vi "导入模版文件.vi"(8 "功率控制表":refnum<vi>, 9 "标定参数表":refnum<vi>, 11 "该应用程序":refnum<vi>) -> ()   [LabVIEW 2015]
uses:
  <vilib>/addons/_office/excel.llb/Excel Get Data ([str]).vi
  <vilib>/Utility/NIReport.llb/NI_report.lvclass
  <vilib>/Utility/NIReport.llb/Excel/NI_Excel.lvclass
  <vilib>/addons/_office/NI_ReportGenerationToolkit.lvlib
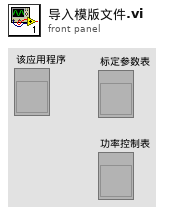
[diagram p1: front panel]
types:
  T1 = enum16{"Standard Report", "HTML", "Word", "Excel"}
  T2 = enum16{"maximized", "minimized", "normal", "no change"}
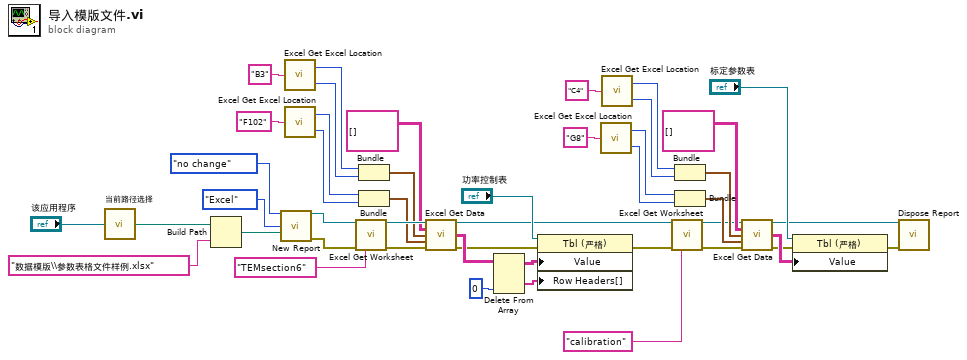
[diagram p0: block diagram]
diagram:
  n1 = call "当前路径选择.vi"("本应用程序"="该应用程序") -> ("当前路径"=w29:path)
  n2 = Build Path(base path=w29, name or relative path="数据模版\\参数表格文件样例.xlsx" ("名称或相对路径")) -> (appended path=w28:path)
  n3 = call <vilib>:"New Report.vi"("window state (normal)"=T2."no change", "report type"=T1."Excel", "template (empty)"=w28) -> ("report out"=w27:refnum<class "NI_report.lvclass">, "error out"=w26:errorcluster)  [unwired: 11 in]
  n4 = call <vilib>:"Excel Get Excel Location.vi"("cell's name"="B3") -> ("row"=w20:i32, "column"=w19:i32)
  n5 = call <vilib>:"Excel Get Excel Location.vi"("cell's name"="F102") -> ("row"=w17:i32, "column"=w16:i32)
  n6 = call <vilib>:"Excel Get Worksheet.vi"("report in"=w27, "error in (no error)"=w26, "name (\"\")"="TEMsection6" ("name (\"\")")) -> ("report out"=w23:refnum<class "NI_report.lvclass">, "error out"=w24:errorcluster)  [unwired: 11 in]
  n7 = Bundle("row"=w20, "column"=w19) -> (w18:cluster{"row":i32, "column":i32})  [unwired: 1 in]
  n8 = Bundle("row"=w17, "column"=w16) -> (w15:cluster{"row":i32, "column":i32})  [unwired: 1 in]
  n9 = call-poly <vilib>:"Excel Get Data.vi"("report in"=w23, "data type"=string[][] [], "start (-1, -1)"=w18, "end (-1, -1)"=w15, "error in (no error)"=w24) -> ("report out"=w8:refnum<class "NI_report.lvclass">, "data"=w12:string[][], "error out"=w4:errorcluster)  [unwired: 8 in]
  n10 = Delete From Array(array=w12, index (col)=0 ("禁用的索引 (列)")) -> (deleted portion=w9:string[], array with subset deleted=w10:string[][])  [unwired: 2 in]
  n11 = property class="Tbl (严格)"(reference="功率控制表", error in=w4, "Value"=w10, "Row Headers[]"=w9) -> (error out=w3:errorcluster)  [unwired: 1 out]
  n12 = call <vilib>:"Excel Get Excel Location.vi"("cell's name"="G8") -> ("row"=w42:i32, "column"=w41:i32)
  n13 = call <vilib>:"Excel Get Excel Location.vi"("cell's name"="C4") -> ("row"=w38:i32, "column"=w39:i32)
  n14 = call <vilib>:"Excel Get Worksheet.vi"("report in"=w8, "error in (no error)"=w3, "name (\"\")"="calibration" ("name (\"\")")) -> ("report out"=w35:refnum<class "NI_report.lvclass">, "error out"=w34:errorcluster)  [unwired: 11 in]
  n15 = Bundle("row"=w38, "column"=w39) -> (w40:cluster{"row":i32, "column":i32})  [unwired: 1 in]
  n16 = Bundle("row"=w42, "column"=w41) -> (w44:cluster{"row":i32, "column":i32})  [unwired: 1 in]
  n17 = call-poly <vilib>:"Excel Get Data.vi"("report in"=w35, "data type"=string[][] [], "start (-1, -1)"=w40, "end (-1, -1)"=w44, "error in (no error)"=w34) -> ("report out"=w5:refnum<class "NI_report.lvclass">, "data"=w45:string[][], "error out"=w2:errorcluster)  [unwired: 8 in]
  n18 = property class="Tbl (严格)"(reference="标定参数表", error in=w2, "Value"=w45) -> (error out=w1:errorcluster)  [unwired: 1 out]
  n19 = call-dynamic "Dispose Report.vi"("report in"=w5, "error in (no error)"=w1) -> ()  [unwired: 13 in, 1 out]
